vi "PID - Tool.vi"() -> ()   [LabVIEW 2013, in "PID Control Workspace Tool.lvlib"]
uses:
  PID Control Workspace Tool.lvlib
  NationalInstruments.VeriStand.SystemStorage
  Shared/Types/Get Settings Message.ctl
  Shared/Types/Gain Schedule.ctl
  Shared/Types/Update Parameters Message.ctl
  Host API/PID Control Host API.lvlib
  Shared/Control Addon Shared.lvlib
  <vilib>/NI Veristand/Execution/Workspace/NI_VS Workspace ExecutionAPI.lvlib
  <vilib>/NI VeriStand/Execution/CustomDevice/NI_VS Custom Device ExecutionAPI.lvlib
panel:
  in  "NIVS.Gateway IP Address":string
  out "Gain Scheduling Allowed?":bool
  in  "Reset":bool
  in  "Apply":bool
  out "Live Updates Allowed?":bool
  in  "PID Controller Name":u16(ring)
  in  "PID Settings":i32(listbox)
  in  "NIVS.System Definition Root":refnum<k24>
  out "Device":string
  in  "NIVS.Workspace Event":refnum<event-registration>
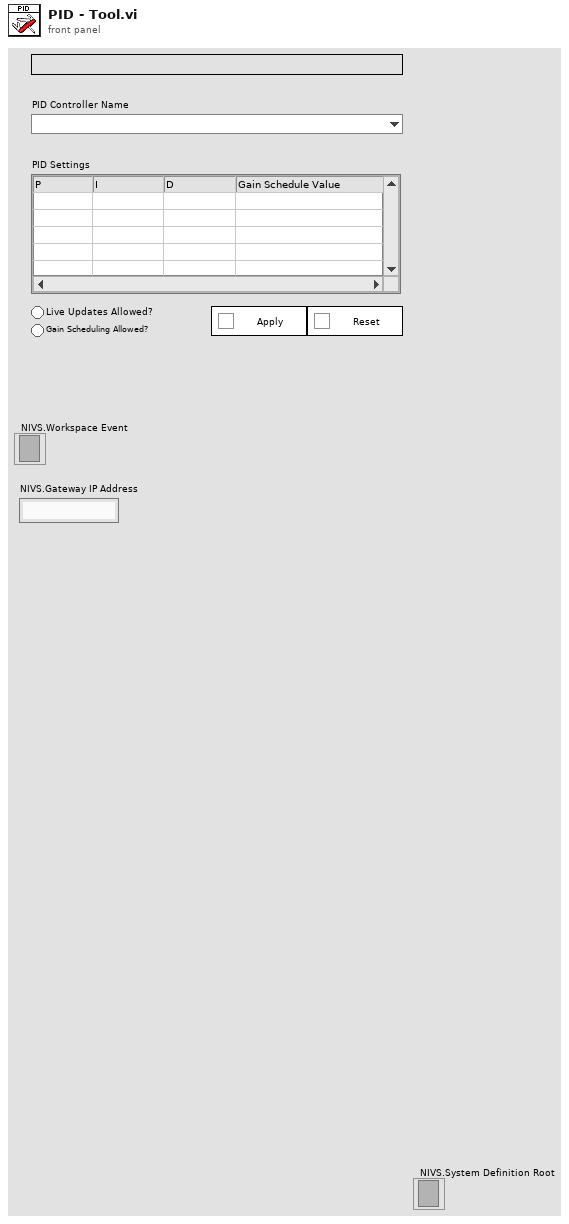
[diagram p1: front panel]
types:
  T1 = typedef "Control Addon Shared.lvlib/Get Settings Message.ctl" = cluster{"Control Loop Names":string[], "Enable Live Updates":bool[], "Gain Schedule":T2[], "Enable Gain Scheduling":bool[]}
  T2 = typedef "Control Addon Shared.lvlib/Gain Schedule.ctl" = cluster{"Gain Schedule":cluster{"PID gains":cluster{"proportional gain (Kc)":dbl, "integral time (Ti, min)":dbl, "derivative time (Td, min)":dbl}, "max value":dbl}[]}
  T3 = cluster{"CD Path":string, "CD IP":string, "Settings":T1}
  T4 = typedef "NI_VS Workspace ExecutionAPI.lvlib/WorkspaceAPI.ctl" = refnum<k24>
  T5 = typedef "NI_VS Workspace ExecutionAPI.lvlib/SystemStateEventRef.ctl" = cluster{"CustDatRef":refnum<user-event>, "EvtRef":refnum<k27>}
  T6 = typedef "NI_VS Workspace ExecutionAPI.lvlib/SystemStateRegEventRef.ctl" = refnum<event-registration>
  T7 = cluster{"NIVS.Workspace Event":refnum<event-registration>, "SystemChangeEventRef":T6}
  T8 = typedef "Control Addon Shared.lvlib/Update Parameters Message.ctl" = cluster{"Control Loop":string, "Gain Schedule":cluster{"PID gains":cluster{"proportional gain (Kc)":dbl, "integral time (Ti, min)":dbl, "derivative time (Td, min)":dbl}, "max value":dbl}[]}
  T9 = typedef "NI_VS Workspace ExecutionAPI.lvlib/SystemState.ctl" = u8
  T10 = cluster{"PID gains":cluster{"proportional gain (Kc)":dbl, "integral time (Ti, min)":dbl, "derivative time (Td, min)":dbl}, "max value":dbl}[]
  T11 = typedef "NI_VS Custom Device ExecutionAPI.lvlib/Custom Device Ref.ctl" = refnum<k24>
  T12 = cluster{"proportional gain (Kc)":dbl, "integral time (Ti, min)":dbl, "derivative time (Td, min)":dbl}
  T13 = typedef "LVPoint32TypeDef.ctl" = cluster{"Horizontal":i32, "Vertical":i32}
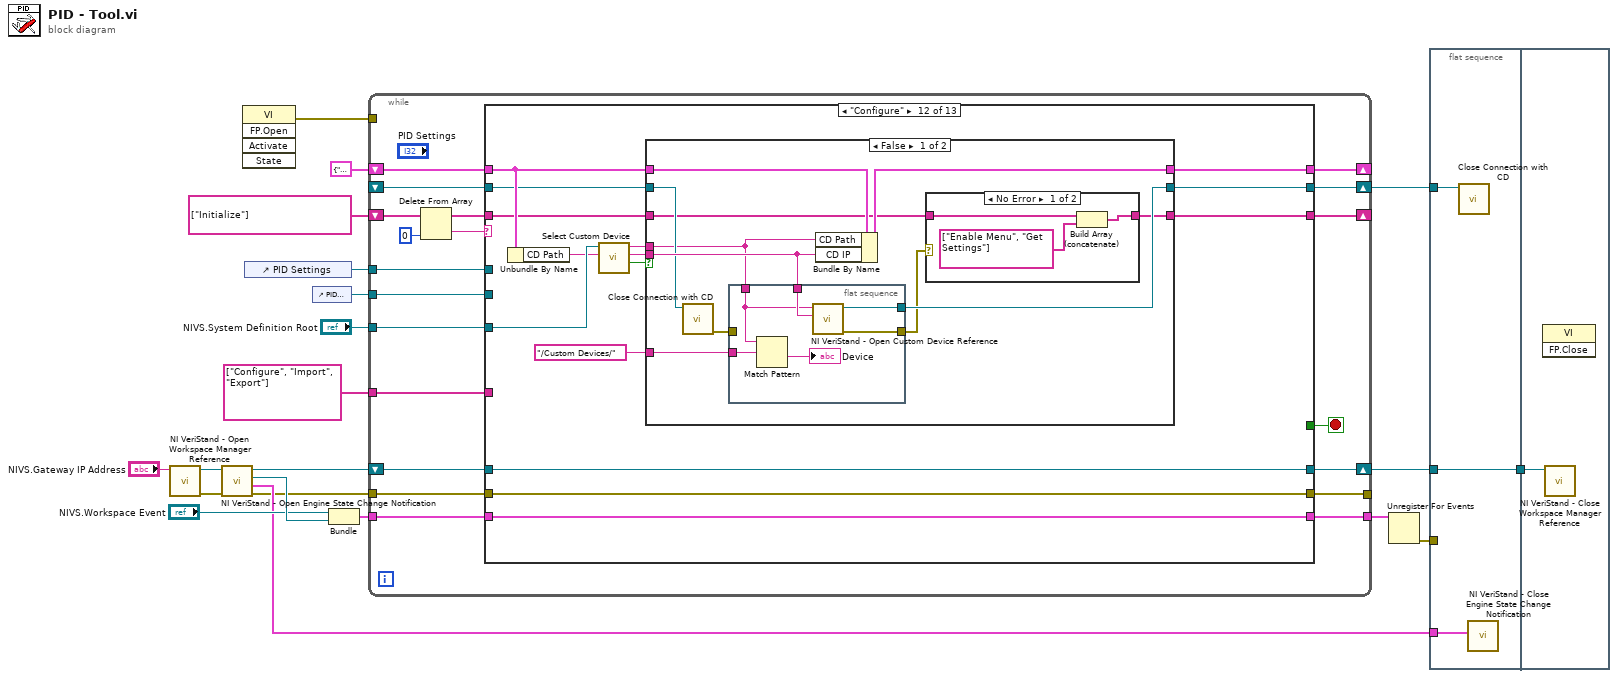
[diagram p0: block diagram]
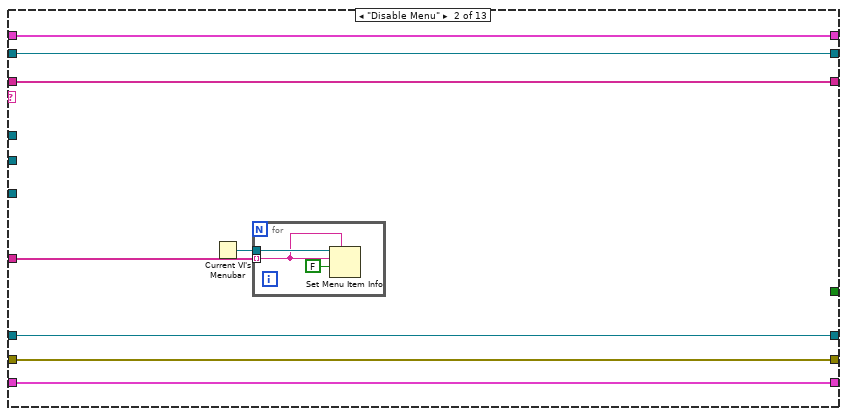
[diagram p3: hidden frame]
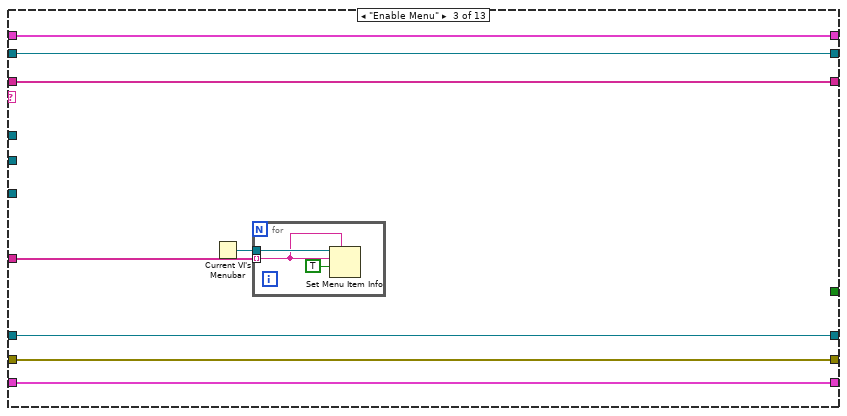
[diagram p4: hidden frame]
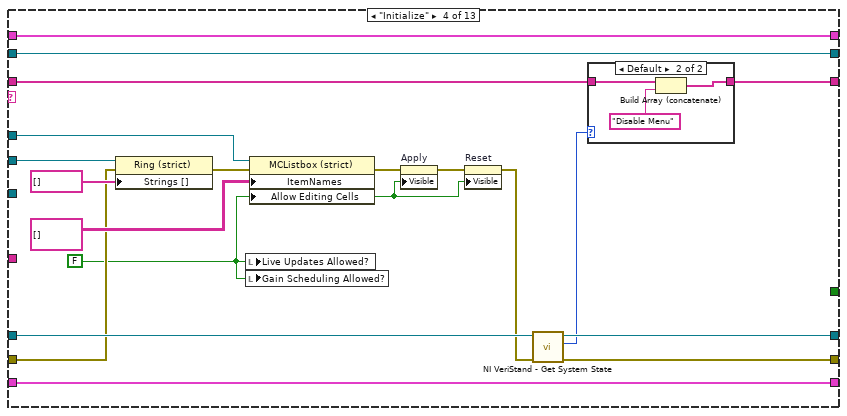
[diagram p5: hidden frame]
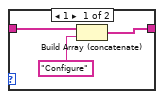
[diagram p6: hidden frame]
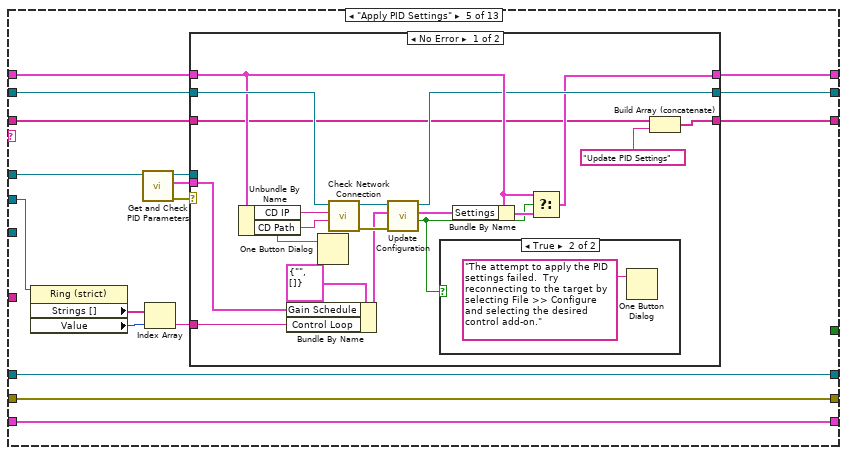
[diagram p7: hidden frame]
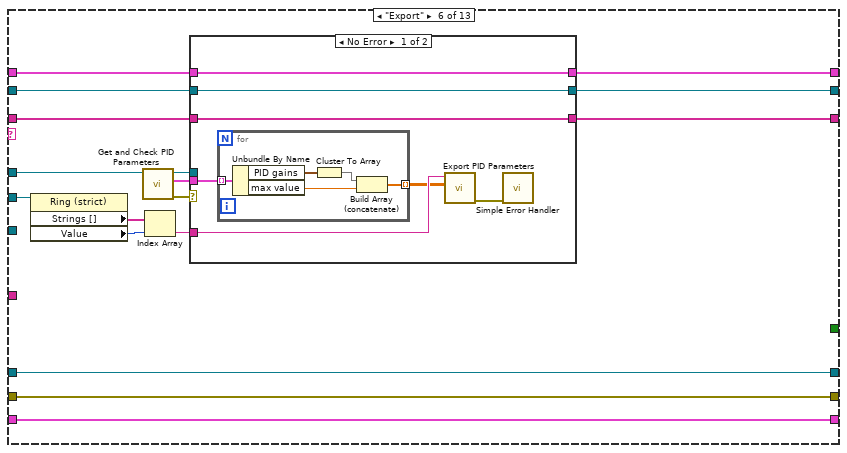
[diagram p10: hidden frame]
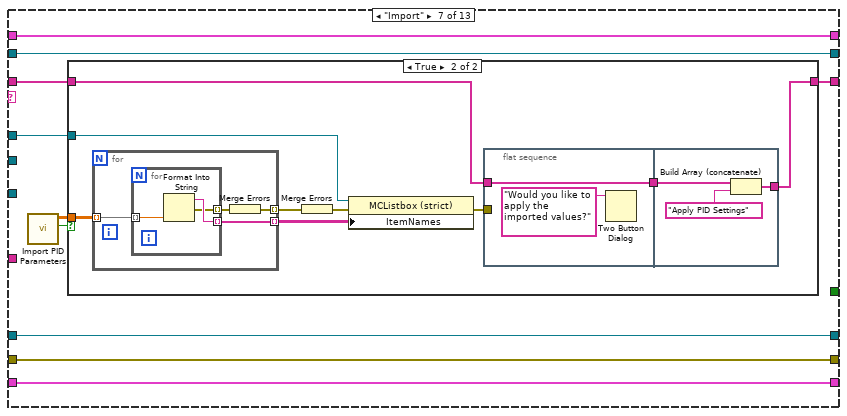
[diagram p12: hidden frame]
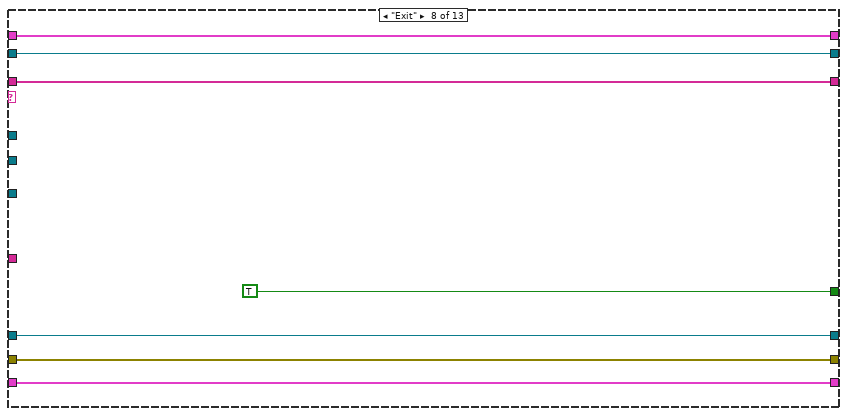
[diagram p14: hidden frame]
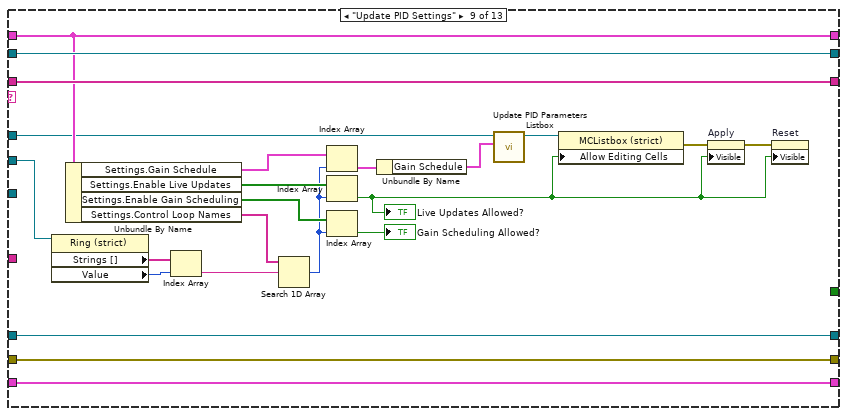
[diagram p15: hidden frame]
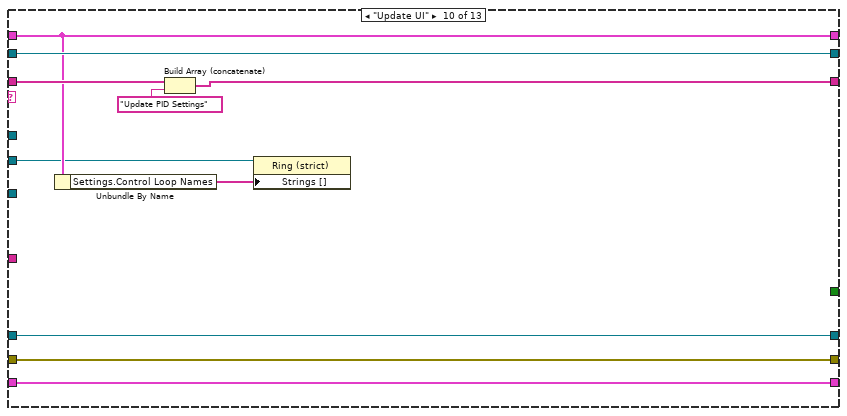
[diagram p16: hidden frame]
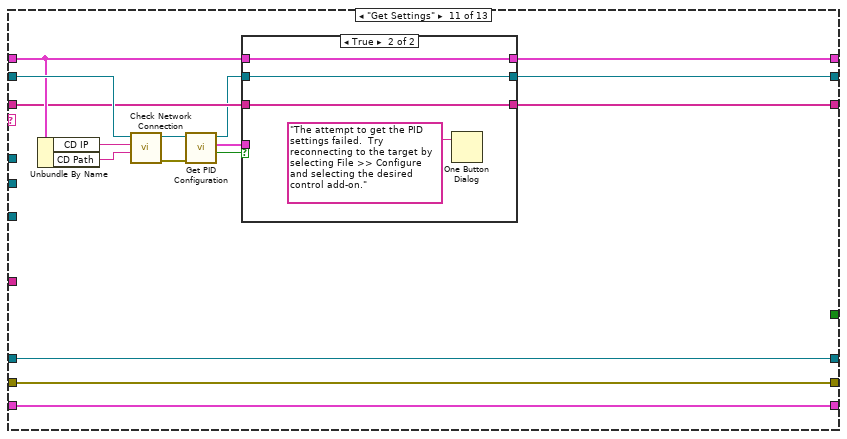
[diagram p17: hidden frame]
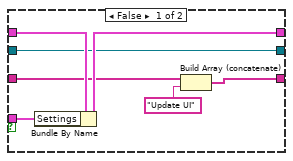
[diagram p18: hidden frame]
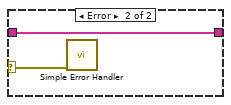
[diagram p19: hidden frame]
diagram:
  n1 = call <vilib>:"NI VeriStand - Open Workspace Manager Reference.vi"("Gateway IP Address (\"\": localhost)"="NIVS.Gateway IP Address") -> ("error out"=w13:errorcluster, "WorkspaceManager"=w14:T4)  [unwired: 9 in]
  n2 = call <vilib>:"NI VeriStand - Open Engine State Change Notification.vi"("error in (no error)"=w13, "WorkspaceManager in"=w14) -> ("error out"=w4:errorcluster, "SystemStateRefs"=w9:T5, "SystemChangeEventRef"=w12:T6, "WorkspaceManager out"=w5:T4)  [unwired: 6 in]
  n3 = invoke class="VI" method="FP.Open"() -> (error out=w17:errorcluster)  [unwired: 5 in, 4 out]
  n4 = control-ref of="PID Settings"() -> (w16:refnum<vi>)
  n5 = control-ref of="PID Controller Name"() -> (w15:refnum<vi>)
  n6 = Bundle("NIVS.Workspace Event"="NIVS.Workspace Event", "SystemChangeEventRef"=w12) -> (w11:T7)  [unwired: 1 in]
  n7 = while {
    tunnel: [w40] -> w7
    tunnel: "NIVS.System Definition Root" -> [w39]
    shift-right: [w35] -> _
    shift-left: T3 {"CD Path"="", "CD IP"="", "Settings"={"Control Loop Names"=[], "Enable Live Updates"=[], "Gain Schedule"=[], "Enable Gain Scheduling"=[]}} -> [w38]
    shift-right: [w37] -> w20
    shift-left: _ -> [w36]
    shift-right: [w30] -> _
    shift-left: string[] ["Initialize"] -> [w34]
    tunnel: w17 -> [_]
    tunnel: w16 -> [w29]
    tunnel: w15 -> [w28]
    tunnel: w11 -> [w27]
    tunnel: w4 -> [w25]
    shift-right: [w24] -> w3
    shift-left: w5 -> [w26]
    tunnel: [w23] -> _
    tunnel: string[] ["Configure", "Import", "Export"] -> [w22]
    stop <- w41 stop-if-true
    n8 = Delete From Array(array=w34, index=0) -> (deleted portion=w32:string, array with subset deleted=w31:string[])  [unwired: 1 in]
    n9 = case shown="\"Configure\"" w32 {
      tunnel: [_ _ _ _ _ _ _ TRUE ("Discard?") _ _ _ _ _] -> w41
      tunnel: [w46 w54 w65 w87 w111 w150 w173 w203 w226 w236 w253 w269 w317] -> w40
      tunnel: w39 -> [_ _ _ _ _ _ _ _ _ _ _ w279 _]
      tunnel: w38 -> [w45 w53 w64 w70 w109 w148 w171 w202 w224 w234 w247 w278 w316]
      tunnel: [w44 w52 w63 w86 w107 w146 w172 w201 w225 w235 w241 w270 w315] -> w37
      tunnel: w36 -> [w44 w52 w63 w86 w110 w149 w172 w201 w225 w235 w248 w277 w314]
      tunnel: [w45 w53 w64 w70 w106 w145 w171 w202 w224 w234 w246 w271 w313] -> w35
      tunnel: w27 -> [w46 w54 w65 w87 w111 w150 w173 w203 w226 w236 w253 w269 w312]
      tunnel: w31 -> [w47 w55 w66 w88 w104 w143 w169 w204 w227 w237 w243 w268 w311]
      tunnel: [w47 w55 w66 w75 w103 w142 w168 w204 w227 w233 w242 w267 w310] -> w30
      tunnel: w29 -> [_ _ _ w82 w98 w137 w170 _ w216 _ _ _ w309]
      tunnel: w28 -> [_ _ _ w81 w102 w141 _ _ w220 w231 _ _ _]
      tunnel: w26 -> [w43 w51 w62 w85 w96 w135 w167 w199 w206 w229 w239 w266 w308]
      tunnel: w25 -> [w42 w50 w61 w74 w95 w134 w166 w198 w205 w228 w238 w265 w307]
      tunnel: [w43 w51 w62 w84 w96 w135 w167 w199 w206 w229 w239 w266 w305] -> w24
      tunnel: [w42 w50 w61 w83 w95 w134 w166 w198 w205 w228 w238 w265 w306] -> w23
      tunnel: w22 -> [_ w48 w59 _ _ _ _ _ _ _ _ _ _]
      frame Default {
      }
      frame "Disable Menu" {
        n10 = Current VI's Menubar() -> (w49:refnum<k9>)
        n11 = for {
          tunnel: w49 -> [w58]
          tunnel: w48 -> [w56] mode=indexing
          n12 = Set Menu Item Info(7:w56, 9:FALSE ("enabled"), 10:w56, 11:w58) -> ()  [unwired: 3 in, 2 out]
        }
      }
      frame "Enable Menu" {
        n13 = Current VI's Menubar() -> (w60:refnum<k9>)
        n14 = for {
          tunnel: w60 -> [w69]
          tunnel: w59 -> [w67] mode=indexing
          n15 = Set Menu Item Info(7:w67, 9:TRUE ("enabled"), 10:w67, 11:w69) -> ()  [unwired: 3 in, 2 out]
        }
      }
      frame "Initialize" {
        w72 = FALSE ("Allow Editing Cells")
        n16 = property class="Ring (strict)"(reference=w81, error in=w74, "Strings []"=string[] []) -> (error out=w80:errorcluster)  [unwired: 1 out]
        n17 = local write "Live Updates Allowed?"(w72) -> ()
        n18 = local write "Gain Scheduling Allowed?"(w72) -> ()
        n19 = property class="MCListbox (strict)"(reference=w82, error in=w80, "ItemNames"=string[][] [] ("Item Names"), "Allow Editing Cells"=w72) -> (error out=w76:errorcluster)  [unwired: 1 out]
        n20 = property on="Apply" class="Bool"(error in=w76, "Visible"=w72) -> (error out=w77:errorcluster)  [unwired: 1 in, 1 out]
        n21 = property on="Reset" class="Bool"(error in=w77, "Visible"=w72) -> (error out=w73:errorcluster)  [unwired: 1 in, 1 out]
        n22 = call <vilib>:"NI VeriStand - Get System State.vi"("error in (no error)"=w73, "WorkspaceManager in"=w85) -> ("error out"=w83:errorcluster, "System State"=w71:T9, "WorkspaceManager  out"=w84:T4)  [unwired: 5 in, 2 out]
        n23 = case shown="Default" w71 {
          tunnel: w88 -> [w91 w94]
          tunnel: [w90 w93] -> w75
          frame 1 {
            n24 = Build Array (concatenate)(w91, "Configure") -> (w90:string[])
          }
          frame Default {
            n25 = Build Array (concatenate)(w94, "Disable Menu") -> (w93:string[])
          }
        }
      }
      frame "Apply PID Settings" {
        n26 = property class="Ring (strict)"(reference=w102) -> ("Strings []"=w100:string[], "Value"=w101:u16)  [unwired: 1 in, 2 out]
        n27 = call "Get and Check PID Parameters.vi"("MulticolumnListbox in"=w98) -> ("error out"=w105:errorcluster, "PID Parameters"=w99:T10, "MulticolumnListbox out"=w97:refnum<vi>)  [unwired: 8 in]
        n28 = Index Array(array=w100, index=w101) -> (element=w108:string)
        n29 = case shown="No Error" w105 {
          tunnel: w110 -> [w127 w132]
          tunnel: w109 -> [w125 w133]
          tunnel: w108 -> [w120 _]
          tunnel: [w119 w132] -> w107
          tunnel: [w118 w133] -> w106
          tunnel: w104 -> [w117 w131]
          tunnel: [w114 w131] -> w103
          tunnel: w97 -> [_ _]
          tunnel: w99 -> [w115 _]
          frame No Error {
            n30 = Unbundle By Name(w125) -> ("CD IP"=w128:string, "CD Path"=w112:string)
            n31 = Bundle By Name(cluster=T8 {"Control Loop"="", "Gain Schedule"=[]} ("Parameters"), "Gain Schedule"=w115, "Control Loop"=w120) -> (w122:T8)
            n32 = One Button Dialog(message=w112) -> ()  [unwired: 1 in, 1 out]
            n33 = call "Check Network Connection.vi"("CD Path"=w112, "IP Address"=w128, "Comm Ref"=w127) -> ("error out"=w124:errorcluster, "Comm Ref"=w126:T11)  [unwired: 7 in]
            n34 = call "Update Configuration.vi"("error in (no error)"=w124, "Parameters"=w122, "Comm Ref"=w126) -> ("Timed Out?"=w116:bool, "GetSettings"=w121:T1, "Comm Ref"=w119:T11)  [unwired: 5 in, 1 out]
            n35 = case shown="True" w116 {
              frame False {
              }
              frame True {
                n36 = One Button Dialog(message="The attempt to apply the PID settings failed.  Try reconnecting to the target by selecting File >> Configure and selecting the desired control add-on.") -> ()  [unwired: 1 in, 1 out]
              }
            }
            n37 = Bundle By Name(cluster=w125, "Settings"=w121) -> (w129:T3)
            n38 = Select(t=w125, s=w116, f=w129) -> (s? t:f=w118:T3)
            n39 = Build Array (concatenate)(w117, "Update PID Settings") -> (w114:string[])
          }
          frame Error {
          }
        }
      }
      frame "Export" {
        n40 = property class="Ring (strict)"(reference=w141) -> ("Strings []"=w139:string[], "Value"=w140:u16)  [unwired: 1 in, 2 out]
        n41 = call "Get and Check PID Parameters.vi"("MulticolumnListbox in"=w137) -> ("error out"=w144:errorcluster, "PID Parameters"=w138:T10, "MulticolumnListbox out"=w136:refnum<vi>)  [unwired: 8 in]
        n42 = Index Array(array=w139, index=w140) -> (element=w147:string)
        n43 = case shown="No Error" w144 {
          tunnel: w149 -> [w157 w164]
          tunnel: w148 -> [w156 w165]
          tunnel: w147 -> [w154 _]
          tunnel: [w157 w164] -> w146
          tunnel: [w156 w165] -> w145
          tunnel: w143 -> [w155 w163]
          tunnel: [w155 w163] -> w142
          tunnel: w136 -> [_ _]
          tunnel: w138 -> [w152 _]
          frame No Error {
            n44 = for {
              tunnel: w152 -> [w162] mode=indexing
              tunnel: [w158] -> w151 mode=indexing
              n45 = Unbundle By Name(w162) -> ("PID gains"=w161:T12, "max value"=w159:dbl)
              n46 = Cluster To Array(cluster=w161) -> (array=w160:dbl[])
              n47 = Build Array (concatenate)(w160, w159) -> (w158:dbl[])
            }
            n48 = call "Export PID Parameters.vi"("Parameters"=w151, "Control Loop"=w154) -> ("error out"=w153:errorcluster)  [unwired: 9 in]
            n49 = call <vilib>:"Simple Error Handler.vi"("error in (no error)"=w153) -> ()  [unwired: 4 in, 5 out]
          }
          frame Error {
          }
        }
      }
      frame "Import" {
        n50 = call "Import PID Parameters.vi"() -> ("Apply?"=w175:bool, "Parameters"=w174:dbl[][])  [unwired: 9 in, 1 out]
        n51 = case shown="True" w175 {
          tunnel: w174 -> [_ w182]
          tunnel: w170 -> [_ w181]
          tunnel: w169 -> [w176 w178]
          tunnel: [w176 w179] -> w168
          frame False {
          }
          frame True {
            n52 = for {
              tunnel: w182 -> [w194] mode=indexing
              tunnel: [w193] -> w185 mode=indexing
              tunnel: [w192] -> w183 mode=indexing
              n53 = for {
                tunnel: w194 -> [w195] mode=indexing
                tunnel: [w197] -> w193 mode=indexing
                tunnel: [w196] -> w191 mode=indexing
                n54 = Format Into String(w195) -> (resulting string=w197:string, error out=w196:errorcluster)  [unwired: 3 in]
              }
              n55 = Merge Errors(w191) -> (w192:errorcluster)
            }
            n56 = Merge Errors(w183) -> (w184:errorcluster)
            n57 = property class="MCListbox (strict)"(reference=w181, error in=w184, "ItemNames"=w185) -> (error out=w180:errorcluster)  [unwired: 1 out]
            n58 = flat-sequence {
              tunnel: w180 -> [_]
              tunnel: w178 -> [w186]
              tunnel: [w186] -> w177
              tunnel: [w189] -> w179
              tunnel: w177 -> [w188]
              frame #0 {
                n59 = Two Button Dialog(message="Would you like to apply the imported values?") -> ()  [unwired: 2 in, 1 out]
              }
              frame #1 {
                n60 = Build Array (concatenate)(w188, "Apply PID Settings") -> (w189:string[])
              }
            }
          }
        }
      }
      frame "Exit" {
      }
      frame "Update PID Settings" {
        n61 = property class="Ring (strict)"(reference=w220) -> ("Strings []"=w219:string[], "Value"=w218:u16)  [unwired: 1 in, 2 out]
        n62 = Unbundle By Name(w224) -> ("Settings.Gain Schedule"=w215:T2[], "Settings.Enable Live Updates"=w222:bool[], "Settings.Enable Gain Scheduling"=w209:bool[], "Settings.Control Loop Names"=w213:string[])
        n63 = Index Array(array=w219, index=w218) -> (element=w223:string)
        n64 = Search 1D Array(1D array=w213, element=w223) -> (index of element=w208:i32)  [unwired: 1 in]
        n65 = Index Array(array=w215, index=w208) -> (element=w214:T2)
        n66 = Index Array(array=w222, index=w208) -> (element=w211:bool)
        "Live Updates Allowed?" <- w211
        n67 = Index Array(array=w209, index=w208) -> (element=→"Gain Scheduling Allowed?":bool)
        n68 = Unbundle By Name(w214) -> ("Gain Schedule"=w217:T10)
        n69 = call "Update PID Parameters Listbox.vi"("Gain Schedule"=w217, "MulticolumnListbox in"=w216) -> ("MulticolumnListbox out"=w212:refnum<vi>)  [unwired: 9 in]
        n70 = property class="MCListbox (strict)"(reference=w212, "Allow Editing Cells"=w211) -> (error out=w210:errorcluster)  [unwired: 1 in, 1 out]
        n71 = property on="Apply" class="Bool"(error in=w210, "Visible"=w211) -> (error out=w221:errorcluster)  [unwired: 1 in, 1 out]
        n72 = property on="Reset" class="Bool"(error in=w221, "Visible"=w211) -> ()  [unwired: 1 in, 2 out]
      }
      frame "Update UI" {
        n73 = Unbundle By Name(w234) -> ("Settings.Control Loop Names"=w230:string[])
        n74 = Build Array (concatenate)(w237, "Update PID Settings") -> (w233:string[])
        n75 = property class="Ring (strict)"(reference=w231, "Strings []"=w230) -> ()  [unwired: 1 in, 2 out]
      }
      frame "Get Settings" {
        n76 = Unbundle By Name(w247) -> ("CD IP"=w252:string, "CD Path"=w251:string)
        n77 = call "Check Network Connection.vi"("CD Path"=w251, "IP Address"=w252, "Comm Ref"=w248) -> ("error out"=w250:errorcluster, "Comm Ref"=w249:T11)  [unwired: 7 in]
        n78 = call "Get PID Configuration.vi"("error in (no error)"=w250, "Comm Ref"=w249) -> ("Timed Out?"=w244:bool, "Settings"=w245:T1, "Comm Ref"=w240:T11)  [unwired: 6 in, 1 out]
        n79 = case shown="True" w244 {
          tunnel: w247 -> [w260 w263]
          tunnel: [w259 w263] -> w246
          tunnel: w245 -> [w258 _]
          tunnel: w243 -> [w257 w264]
          tunnel: [w255 w264] -> w242
          tunnel: [w254 w262] -> w241
          tunnel: w240 -> [w254 w262]
          frame False {
            n80 = Bundle By Name(cluster=w260, "Settings"=w258) -> (w259:T3)
            n81 = Build Array (concatenate)(w257, "Update UI") -> (w255:string[])
          }
          frame True {
            n82 = One Button Dialog(message="The attempt to get the PID settings failed.  Try reconnecting to the target by selecting File >> Configure and selecting the desired control add-on.") -> ()  [unwired: 1 in, 1 out]
          }
        }
      }
      frame "Configure" {
        n83 = Unbundle By Name(w278) -> ("CD Path"=w276:string)
        n84 = call "Select Custom Device.vi"("CD Path"=w276, "NIVS.System Definition Root"=w279) -> ("Cancelled?"=w275:bool, "IP Address"=w274:string, "Custom Device Path Out"=w273:string)  [unwired: 7 in]
        n85 = case shown="False" w275 {
          tunnel: w274 -> [w288 _]
          tunnel: w273 -> [w280 _]
          tunnel: "/Custom Devices/" ("regular expression") -> [w290 _]
          tunnel: w278 -> [w289 w303]
          tunnel: [w287 w304] -> w270
          tunnel: w277 -> [w286 w304]
          tunnel: [w285 w303] -> w271
          tunnel: w268 -> [w284 w302]
          tunnel: [w282 w302] -> w267
          frame False {
            n86 = call "Close Connection with CD.vi"("Comm Ref"=w286) -> ("error out"=w281:errorcluster)  [unwired: 10 in]
            n87 = flat-sequence {
              tunnel: w290 -> [w296]
              tunnel: w280 -> [w293]
              tunnel: w288 -> [w294]
              tunnel: [w292] -> w287
              tunnel: [w291] -> w283
              tunnel: w281 -> [_]
              frame #0 {
                n88 = Match Pattern(string=w293, regular expression=w296) -> (after substring=→"Device":string)  [unwired: 1 in, 3 out]
                n89 = call <vilib>:"NI VeriStand - Open Custom Device Reference.vi"("Gateway IP Address (\"\": localhost)"=w294, "Custom Device Path"=w293) -> ("error out"=w291:errorcluster, "Custom Device"=w292:T11)  [unwired: 8 in]
              }
            }
            n90 = Bundle By Name(cluster=w289, "CD Path"=w280, "CD IP"=w288) -> (w285:T3)
            n91 = case shown="No Error" w283 {
              selector: w283 -> [_ w300]
              tunnel: w284 -> [w299 w301]
              tunnel: [w298 w301] -> w282
              frame No Error {
                n92 = Build Array (concatenate)(w299, string[] ["Enable Menu", "Get Settings"]) -> (w298:string[])
              }
              frame Error {
                n93 = call <vilib>:"Simple Error Handler.vi"("error in (no error)"=w300) -> ()  [unwired: 4 in, 5 out]
              }
            }
          }
          frame True {
          }
        }
      }
      frame "" {
        n94 = event shown="[5] \"Apply\": Value Change" {
          selector: w312 -> [_ _ _ _ _ _ _ _ _]
          dyn-events: [_ _ _ _ _ _ _ _ _] -> w317
          timeout: _ -> [_ _ _ _ _ _ _ _ _]
          tunnel: w316 -> [w321 w329 w337 w345 w366 w375 w385 w393 w413]
          tunnel: [w322 w330 w338 w344 w367 w376 w386 w401 w414] -> w315
          tunnel: w314 -> [w322 w330 w338 w344 w367 w376 w386 w401 w414]
          tunnel: [w321 w329 w337 w345 w366 w375 w385 w393 w413] -> w313
          tunnel: w311 -> [w324 w331 w336 w352 w365 w379 w384 w395 w411]
          tunnel: [w320 w328 w335 w352 w365 w378 w383 w394 w410] -> w310
          tunnel: w309 -> [_ _ _ _ w361 _ _ _ _]
          tunnel: w308 -> [w319 w326 w333 w340 w360 w374 w381 w400 w409]
          tunnel: w307 -> [w318 w325 w332 w339 w359 w373 w380 w399 w408]
          tunnel: [w318 w325 w332 w339 w359 w373 w380 w398 w408] -> w306
          tunnel: [w319 w326 w333 w340 w360 w374 w381 w397 w409] -> w305
          event Menu Selection (User) {
            n95 = event-data() -> ("ItemTag"=w323:string)  [unwired: 1 out]
            n96 = Build Array (concatenate)(w324, w323) -> (w320:string[])
          }
          event "PID Controller Name": Value Change {
            n97 = event-data() -> ()  [unwired: 2 out]
            n98 = Build Array (concatenate)(w331, "Update PID Settings") -> (w328:string[])
          }
          event "Reset": Value Change {
            n99 = event-data() -> ()  [unwired: 3 out]
            n100 = Build Array (concatenate)(w336, "Update PID Settings") -> (w335:string[])
          }
          event "PID Settings": Shortcut Menu Activation? {
            n101 = event-data() -> ("MenuRef"=w351:refnum<k9>, "CtlRef"=w348:refnum<vi>, "Coords"=w347:T13)  [unwired: 1 out]
            n102 = local read "Gain Scheduling Allowed?"() -> (w343:bool)
            n103 = local read "Live Updates Allowed?"() -> (w341:bool)
            n104 = Delete Menu Items(9:w351) -> (0:w349:errorcluster, 3:w350:refnum<k9>)  [unwired: 3 in]
            n105 = Compound Arithmetic op=AND(w343, w341) -> (w342:bool)
            n106 = case shown="True" w342 {
              tunnel: w348 -> [_ w358]
              tunnel: w347 -> [_ w357]
              tunnel: w350 -> [_ w356]
              tunnel: [w353 w355] -> _
              tunnel: w349 -> [w353 w354]
              frame False {
              }
              frame True {
                n107 = call "Manage Menu Items.vi"("error in (no error)"=w354, "Coords"=w357, "CtlRef"=w358, "Menu in"=w356) -> ("error out"=w355:errorcluster)  [unwired: 7 in]
              }
            }
            n108 = event-data("Discard?"=FALSE) -> ()  [unwired: 1 in, 1 out]
          }
          event "PID Settings": Shortcut Menu Selection (User) {
            n109 = event-data() -> ("ItemTag"=w362:string, "CtlRef"=w363:refnum<vi>, "Coords"=w364:T13)  [unwired: 1 out]
            n110 = case shown="\"Delete Row\"" w362 {
              tunnel: w361 -> [_ _ w372]
              tunnel: [_ w368 w371] -> _
              tunnel: w363 -> [_ w370 _]
              tunnel: w364 -> [_ w369 _]
              frame Default {
              }
              frame "Delete Row" {
                n111 = call "Delete PID Parameter Row.vi"("Coords"=w369, "MulticolumnListbox in"=w370) -> ("error out"=w368:errorcluster)  [unwired: 9 in]
              }
              frame "Add Row" {
                n112 = call "Add PID Parameter Row.vi"("MulticolumnListbox in"=w372) -> ("error out"=w371:errorcluster)  [unwired: 10 in]
              }
            }
          }
          event "Apply": Value Change {
            n113 = event-data() -> ()  [unwired: 3 out]
            n114 = Build Array (concatenate)(w379, "Apply PID Settings") -> (w378:string[])
          }
          event User Event {
            n115 = event-data() -> ("Workspace Event"=w387:string)  [unwired: 1 out]
            n116 = Equal?(x=w387, y="Shut Down") -> (x = y?=w382:bool)
            n117 = case shown="True" w382 {
              tunnel: w384 -> [w389 w392]
              tunnel: [w389 w390] -> w383
              frame False {
              }
              frame True {
                n118 = Build Array (concatenate)(w392, "Exit" ("y")) -> (w390:string[])
              }
            }
          }
          event User Event {
            n119 = event-data() -> ()  [unwired: 2 out]
            n120 = call <vilib>:"NI VeriStand - Get System State.vi"("error in (no error)"=w399, "WorkspaceManager in"=w400) -> ("error out"=w398:errorcluster, "System State"=w396:T9, "WorkspaceManager  out"=w397:T4)  [unwired: 5 in, 2 out]
            n121 = case shown="0, Default" w396 {
              tunnel: w395 -> [w404 w407]
              tunnel: [w403 w406] -> w394
              frame 0, Default {
                n122 = Build Array (concatenate)(w404, "Initialize") -> (w403:string[])
              }
              frame 1 {
                n123 = Build Array (concatenate)(w407, "Configure") -> (w406:string[])
              }
            }
          }
          event Panel Close? {
            n124 = event-data() -> ()  [unwired: 5 out]
            n125 = Build Array (concatenate)(w411, "Exit" ("y")) -> (w410:string[])
            n126 = event-data("Discard?"=TRUE) -> ()  [unwired: 1 in, 1 out]
          }
        }
      }
    }
  }
  n127 = Unregister For Events(event registration refnum=w7) -> (error out=w6:errorcluster)  [unwired: 1 in]
  n128 = flat-sequence {
    tunnel: w20 -> [w418]
    tunnel: w9 -> [w417]
    tunnel: [w416] -> w8
    tunnel: w3 -> [w416]
    tunnel: w6 -> [_]
    tunnel: w8 -> [w419]
    frame #0 {
      n129 = call "Close Connection with CD.vi"("Comm Ref"=w418) -> ()  [unwired: 10 in, 1 out]
      n130 = call <vilib>:"NI VeriStand - Close Engine State Change Notification.vi"("SystemStateRefs"=w417) -> ()  [unwired: 10 in, 1 out]
    }
    frame #1 {
      n131 = invoke class="VI" method="FP.Close"() -> ()  [unwired: 3 in, 3 out]
      n132 = call <vilib>:"NI VeriStand - Close Workspace Manager Reference.vi"("WorkspaceManager"=w419) -> ()  [unwired: 10 in, 1 out]
    }
  }
